vi "ATF-Pump-AI Cumulative Sequence Check.vi"(5 "output cluster":T1, 9 "CDT":dbl, 10 "Loop no":i32) -> (1 "Failure case Seq":string, 2 "Boolean":bool, 3 "String":string)   [LabVIEW 2022 SP3]
uses:
  RT Controls/ATF-Pump-FGV Read write.ctl
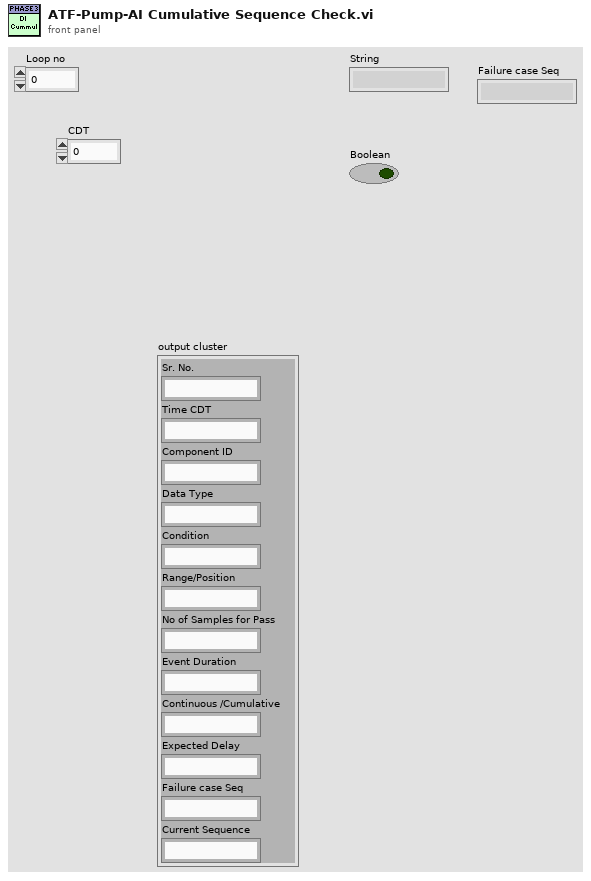
[diagram p1: front panel]
types:
  T1 = cluster{"Sr. No.":string, "Time CDT":string, "Component ID":string, "Data Type":string, "Condition":string, "Range/Position":string, "No of Samples for Pass":string, "Event Duration":string, "Continuous /Cumulative":string, "Expected Delay":string, "Failure case Seq":string, "Current Sequence":string}
  T2 = typedef "ATF-Pump-FGV Read write.ctl" = enum16{"Write", "Read"}
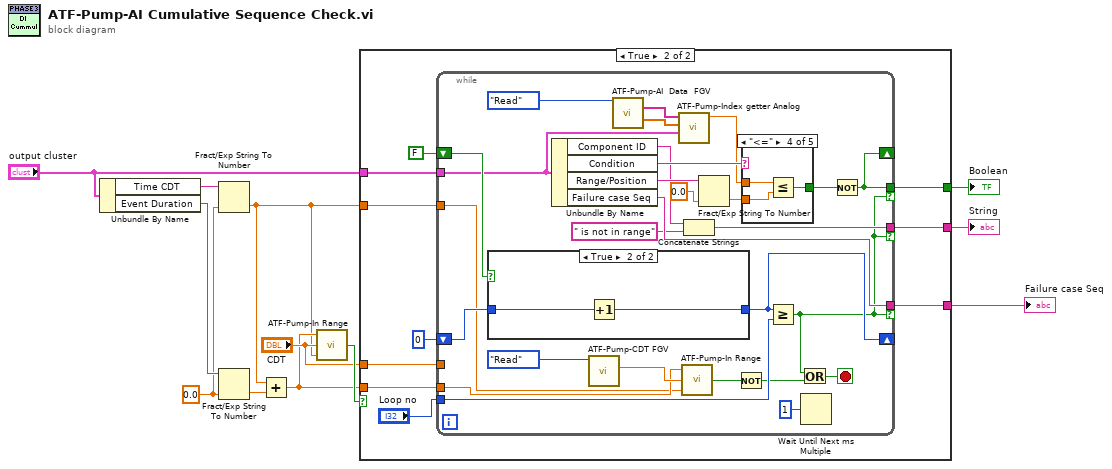
[diagram p0: block diagram]
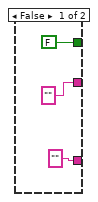
[diagram p2: hidden frame]
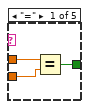
[diagram p3: hidden frame]
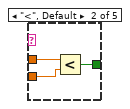
[diagram p4: hidden frame]
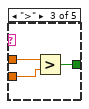
[diagram p5: hidden frame]
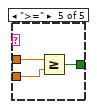
[diagram p6: hidden frame]
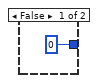
[diagram p7: hidden frame]
diagram:
  w8 = 0.0
  n1 = Unbundle By Name("output cluster") -> ("Time CDT"=w10:string, "Event Duration"=w9:string)
  n2 = Fract/Exp String To Number(string=w10, default (0 dbl)=w8) -> (number=w1:dbl)  [unwired: 2 in, 1 out]
  n3 = Fract/Exp String To Number(string=w9, default (0 dbl)=w8) -> (number=w11:dbl)  [unwired: 2 in, 1 out]
  n4 = Add(x=w1, y=w11) -> (x+y=w2:dbl)
  n5 = call "ATF-Pump-In Range.vi"("Min"=w1, "X"="CDT", "Max"=w2) -> ("In Range"=w7:bool)  [unwired: 2 in]
  n6 = case shown="True" w7 {
    tunnel: "output cluster" -> [_ w24]
    tunnel: "CDT" -> [_ w23]
    tunnel: [FALSE w22] -> w6
    tunnel: ["" w21] -> w5
    tunnel: ["" ("Failure case Seq") w20] -> w4
    tunnel: w2 -> [_ w17]
    tunnel: w1 -> [_ w16]
    frame False {
    }
    frame True {
      n7 = while {
        tunnel: w24 -> [w27]
        tunnel: [w50] -> w21 if=w34
        shift-right: [w45] -> _
        shift-left: FALSE -> [w48]
        shift-right: [w47] -> _
        shift-left: 0 ("Numeric") -> [w49]
        tunnel: [w46] -> w20 if=w34
        tunnel: [w45] -> w22 if=w34
        tunnel: w23 -> [_]
        tunnel: "Loop no" -> [w40]
        tunnel: w17 -> [w33]
        tunnel: w16 -> [w32]
        stop <- w35 stop-if-true
        n8 = case shown="True" w48 {
          tunnel: [0 w71] -> w47
          tunnel: w49 -> [_ w70]
          frame False {
          }
          frame True {
            n9 = Increment(x=w70) -> (x+1=w71:i32)
          }
        }
        n10 = Unbundle By Name(w27) -> ("Component ID"=w51:string, "Condition"=w52:string, "Range/Position"=w53:string, "Failure case Seq"=w46:string)
        n11 = call "ATF-Pump-CDT FGV.vi"("Write/Read"=enum16{"Write", "Read"}."Read") -> ("CDT Out"=w38:dbl)  [unwired: 9 in, 1 out]
        n12 = call "ATF-Pump-AI  Data  FGV.vi"("Write/Read"=ATF-Pump-FGV_Read_write."Read") -> ("AI Channels Name LP"=w29:string[], "AI Y LP data"=w28:dbl[])  [unwired: 11 in, 2 out]
        n13 = call "ATF-Pump-Index getter Analog.vi"("output cluster"=w27, "AI Y  data"=w28, "AI Channels Name"=w29) -> ("Analog data"=w31:dbl)  [unwired: 8 in]
        n14 = call "ATF-Pump-In Range.vi"("Min"=w32, "X"=w38, "Max"=w33) -> ("In Range"=w36:bool)  [unwired: 2 in]
        n15 = Concatenate Strings(w51, " is not in range" ("string")) -> (w50:string)
        n16 = Fract/Exp String To Number(string=w53, default (0 dbl)=0.0) -> (number=w43:dbl)  [unwired: 2 in, 1 out]
        n17 = Not(x=w36) -> (.not. x?=w37:bool)
        n18 = case shown="\"<=\"" w52 {
          tunnel: w43 -> [w56 w58 w61 w64 w67]
          tunnel: w31 -> [w55 w59 w62 w65 w68]
          tunnel: [w54 w57 w60 w63 w66] -> w41
          frame "=" {
            n19 = Equal?(x=w55, y=w56) -> (x = y?=w54:bool)
          }
          frame "<", Default {
            n20 = Less?(x=w59, y=w58) -> (x < y?=w57:bool)
          }
          frame ">" {
            n21 = Greater?(x=w62, y=w61) -> (0:w60:bool)
          }
          frame "<=" {
            n22 = Less Or Equal?(x=w65, y=w64) -> (x <= y?=w63:bool)
          }
          frame ">=" {
            n23 = Greater Or Equal?(x=w68, y=w67) -> (x >= y?=w66:bool)
          }
        }
        n24 = Greater Or Equal?(x=w47, y=w40) -> (x >= y?=w34:bool)
        n25 = Or(x=w34, y=w37) -> (x .or. y?=w35:bool)
        n26 = Wait Until Next ms Multiple(millisecond multiple=u32 1) -> ()  [unwired: 1 out]
        n27 = Not(x=w41) -> (.not. x?=w45:bool)
      }
    }
  }
  "Failure case Seq" <- w4
  "String" <- w5
  "Boolean" <- w6
